vi "Operator Joystick Controls.vi"(1 "Button 4":bool, 2 "Button 5":bool, 3 "Button 6":bool, 4 "Button 7":bool, 6 "Button 3":bool, 7 "Button 8":bool, 8 "Button 2":bool, 9 "Button 9":bool, 10 "Button 1":bool, 11 "Button 10":bool, 12 "axis 3 (throttle)":dbl, 13 "Button 11":bool) -> ()   [LabVIEW 2013]
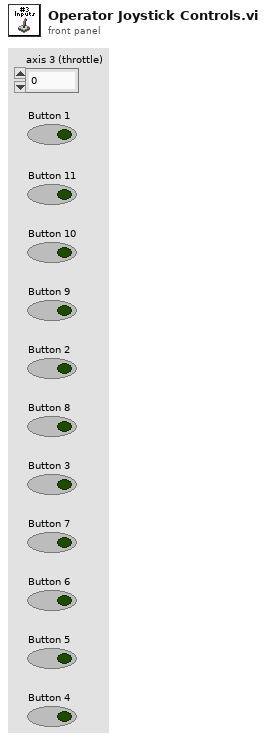
[diagram p1: front panel]
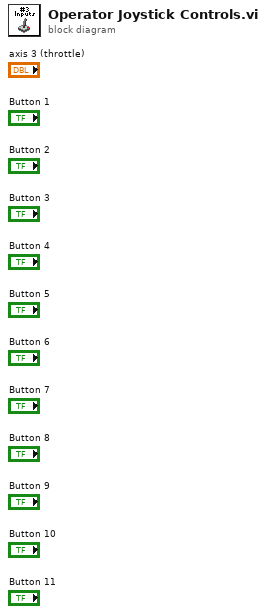
[diagram p0: block diagram]
diagram:
